vi "Convert with Linear Calibration (inverse) (1D, DBL).vi"(10 "Linear Calibration 1D":T1, 11 "A*":dbl) -> (3 "A":dbl)   [LabVIEW 2011, in "COSYLib.lvlib"]
doc: "Calculates X=(Y-B)/A, with A and B taken from a <B>Linear Calibration</B> cluster."
uses:
  COSYLib.lvlib
  Linear Calibration 1D.ctl
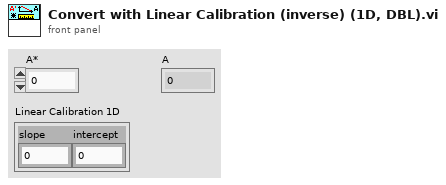
[diagram p1: front panel]
types:
  T1 = typedef "COSYLib.lvlib/Linear Calibration 1D.ctl" = cluster{"slope":dbl, "intercept":dbl}
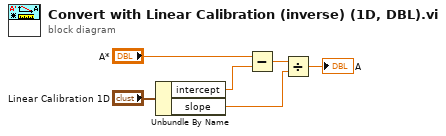
[diagram p0: block diagram]
diagram:
  n1 = Unbundle By Name("Linear Calibration 1D") -> ("intercept"=w4:dbl, "slope"=w2:dbl)
  n2 = Subtract(x="A*", y=w4) -> (x-y=w3:dbl)
  n3 = Divide(x=w3, y=w2) -> (x/y=→"A":dbl)
